vi "Process.vi"(8 "error in":errorcluster, 11 "CAN Task in":refnum<class "CAN Task.lvclass">) -> (0 "error out":errorcluster, 3 "CAN Task out":refnum<class "CAN Task.lvclass">)   [LabVIEW 2024, in "canopen.lvlib" / "CAN Task.lvlib" / "CAN Task.lvclass"]
uses:
  CAN Task.lvclass
  CAN Task.lvclass/CAN Task.ctl
panel:
  out "Processed?":bool
  in  "Value":cluster{"CobID":u32, "nBytes":u8}[](array[cluster])
  in  "Data":u8[](array[numeric])
  in  "COB id":u32 format="%.0x"
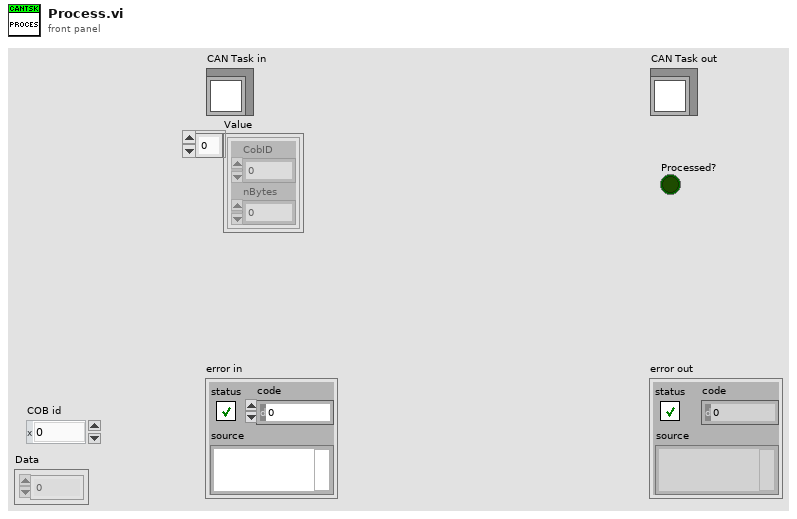
[diagram p1: front panel]
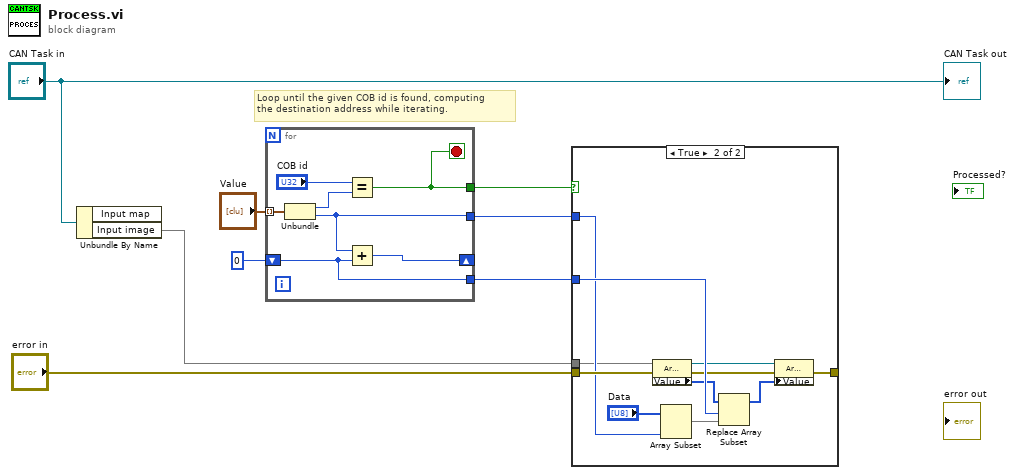
[diagram p0: block diagram]
diagram:
  # "Loop until the given COB id is found, computing\nthe destination address while iterating."
  n1 = Unbundle By Name("CAN Task in") -> ("Input map"=w5, "Input image"=w4)
  n2 = for {
    tunnel: "Value" -> [w16] mode=indexing
    shift-right: [w14] -> _
    shift-left: 0 -> [w13]
    tunnel: [w13] -> w7
    tunnel: [w12] -> w8
    tunnel: [w11] -> w6
    stop <- w12 stop-if-true
    n3 = Unbundle(w16) -> ("CobID"=w15:u32, "nBytes"=w11:u8)
    n4 = Equal?(x="COB id", y=w15) -> (x = y?=w12:bool)
    n5 = Add(x=w11, y=w13) -> (x+y=w14:i32)
  }
  n6 = case shown="True" w8 {
    tunnel: w7 -> [_ w27]
    tunnel: w6 -> [_ w19]
    tunnel: [w17 w21] -> _
    tunnel: "error in" -> [w17 w20]
    tunnel: w4 -> [_ w18]
    frame False {
    }
    frame True {
      n7 = property class="Arr (strict)"(reference=w18, error in=w20) -> (reference out=w23:refnum<vi>, error out=w22:errorcluster, "Value"=w25:u8[])
      n8 = Array Subset(array="Data", length=w19) -> (w26:u8[])  [unwired: 1 in]
      n9 = Replace Array Subset(array=w25, new element=w26, index=w27) -> (w24:u8[])
      n10 = property class="Arr (strict)"(reference=w23, error in=w22, "Value"=w24) -> (error out=w21:errorcluster)  [unwired: 1 out]
    }
  }
  "CAN Task out" <- "CAN Task in"
